vi "Abort Plugin.vi"(6 "timeout (ms)":i32=5000, 8 "error in":errorcluster, 10 "plugin_name":string, 11 "gRPC ID in":T1) -> (0 "error out":errorcluster, 3 "gRPC ID out":T1)   [LabVIEW 2021, in "CIFManagerClientWrapper.lvlib"]
uses:
  CIFManagerClientWrapper.lvlib
  <vilib>/gRPC/LabVIEW gRPC Library/Shared/grpcId.ctl
  CIF_Manager_client/RPC Messages/cif_manager_AbortPluginRequest.ctl
  CIF_Manager_client/CIF_Manager_client.lvlib
  <vilib>/gRPC/LabVIEW gRPC Library/grpc-lvsupport-release.lvlib
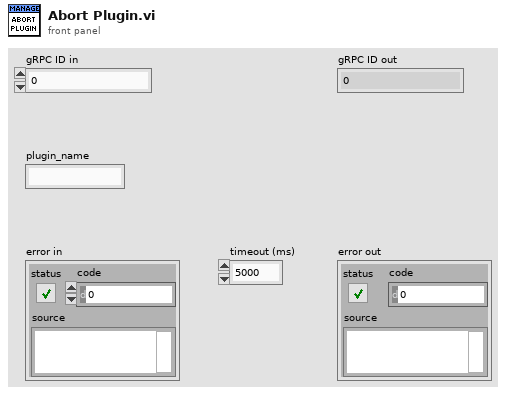
[diagram p1: front panel]
types:
  T1 = typedef "grpc-lvsupport-release.lvlib/grpcId.ctl" = u64
  T2 = typedef "CIF_Manager_client.lvlib/cif_manager_AbortPluginRequest.ctl" = cluster{"plugin_name":string}
  T3 = typedef "CIF_Manager_client.lvlib/cif_manager_AbortPluginResponse.ctl" = cluster{"status":T4}
  T4 = typedef "CIF_Manager_client.lvlib/cif_common_Status.ctl" = cluster{"code":i32, "message":string}
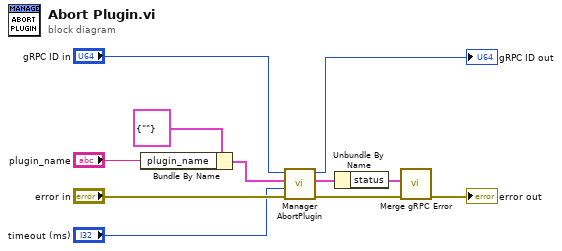
[diagram p0: block diagram]
diagram:
  n1 = Bundle By Name(cluster=T2 {"plugin_name"=""} ("Request Data"), "plugin_name"="plugin_name") -> (w6:T2)
  n2 = call "Manager AbortPlugin.vi"("error in"="error in", "timeout (ms)"="timeout (ms)", "Request Data"=w6, "gRPC ID"="gRPC ID in") -> ("error out"=w5:errorcluster, "Response Data"=w3:T3, "gRPC ID out"=→"gRPC ID out":T1)  [unwired: 5 in]
  n3 = Unbundle By Name(w3) -> ("status"=w1:T4)
  n4 = call "Merge gRPC Error.vi"("error in (no error)"=w5, "gRPC Error"=w1) -> ("error out"=→"error out":errorcluster)  [unwired: 9 in]
